vi "Actor Core.vi"(8 "error in":errorcluster, 11 "KIT-QA in":refnum<class "KIT-QA.lvclass">) -> (0 "error out":errorcluster, 3 "Actor out":refnum<class "Actor.lvclass">)   [LabVIEW 2015, in "KIT-QA.lvlib" / "KIT-QA.lvclass"]
doc: "(<B>Filename</B>: Actor Framework.lvlib:Actor.lvclass:Actor Core.vi)\n\nReceives messages to the actor, reacts to them, and initiates any error handling that may shut the actor down.\n\nDescendant classes may override this VI to append parallel tasks for the actor to complete while it handles messages. Overrides use the Call Parent Method node."
uses:
  KIT-QA.lvclass
  <vilib>/ActorFramework/Actor/Actor.lvclass
  CSPP_Core/Actors/CS++BaseActor/CS++BaseActor.lvclass/CS++BaseActor.ctl
  KIT-QA.lvclass/KIT-QA.ctl
  CSPP_Core/Actors/CS++GUIActor/CS++GUIActor.lvclass/CS++GUIActor.ctl
  <vilib>/ActorFramework/Actor/Actor.lvclass/Actor.ctl
  <vilib>/ActorFramework/Message Enqueuer/Message Enqueuer.lvclass/Message Enqueuer.ctl
  KIT-QA Messages/Save to TDMS Msg/Save to TDMS Msg.lvclass/Save to TDMS Msg.ctl
  KIT-QA Messages/Read QDEvent Logfile Msg/Read QDEvent Logfile Msg.lvclass/Read QDEvent Logfile Msg.ctl
  CSPP_Core/Actors/CS++BaseActor/Read Object Name.vi
  CSPP_Core/Actors/CS++GUIActor/Read Stop-Event.vi
  CSPP_Core/Actors/CS++GUIActor/Read PV-Update.vi
  <vilib>/ActorFramework/Message Enqueuer/Init from Existing Queue.vi
  <vilib>/ActorFramework/Message Enqueuer/Enqueue.vi
  <vilib>/ActorFramework/Message Priority Queue/Priority Enqueue.vi
  <vilib>/Waveform/WDTOps.llb/WDT Waveform Duration DBL.vi
  CSPP_Core/Classes/CS++ProcessVariables/ProcessVariable/PV.lvclass
  <vilib>/ActorFramework/Message Enqueuer/Message Enqueuer.lvclass
  <vilib>/ActorFramework/Stop Msg/Stop Msg.lvclass
  KIT-QA Messages/Save to TDMS Msg/Save to TDMS Msg.lvclass
  KIT-QA Messages/Read QDEvent Logfile Msg/Read QDEvent Logfile Msg.lvclass
  CSPP_Core/Actors/CS++GUIActor/CS++GUIActor.lvclass
  CSPP_Core/Actors/CS++BaseActor/CS++BaseActor.lvclass
  CSPP_Core/Libraries/Utilities/CS++Utilities.lvlib
panel:
  out "Enabled Plots":bool[](array[boolean])
  out "CursLoc":cluster{"X":dbl, "Y":dbl}
  out "Quench Channel":i32
  out "Quench Event Logfile Content":string
  in  "Stop Button":bool
  out "Mixed Signal Graph":T1(graph)
  out "Trace Graph":T2(graph)
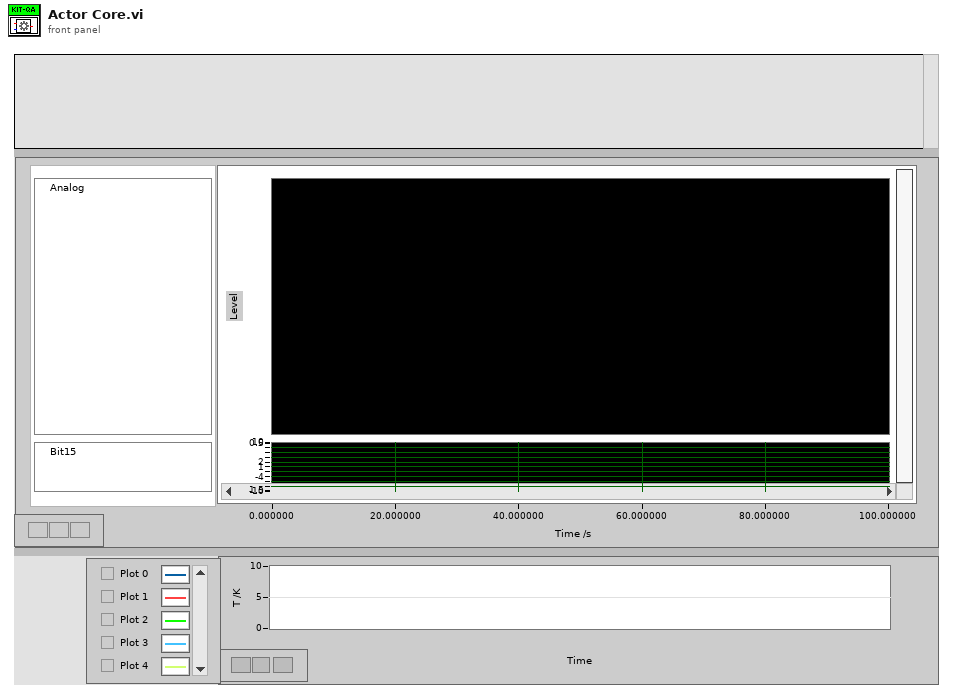
[diagram p1: front panel]
types:
  T1 = cluster{"Analog Wfm":waveform(dbl)[], "Bit 15":digitalwaveform}
  T2 = cluster{"timestamps":timestamp[], "data":dbl[]}[]
  T3 = enum32{"Invalid", "Standard", "Closed", "Hidden", "Minimized", "Maximized"}
  T4 = cluster{"Quench Offset":dbl[unit], "Quench Channel":i32, "Bit 15":digitalwaveform, "Analog Wfm":waveform(dbl)[]}
  T5 = enum8{"Enabled", "Disabled", "Disabled and Grayed Out"}
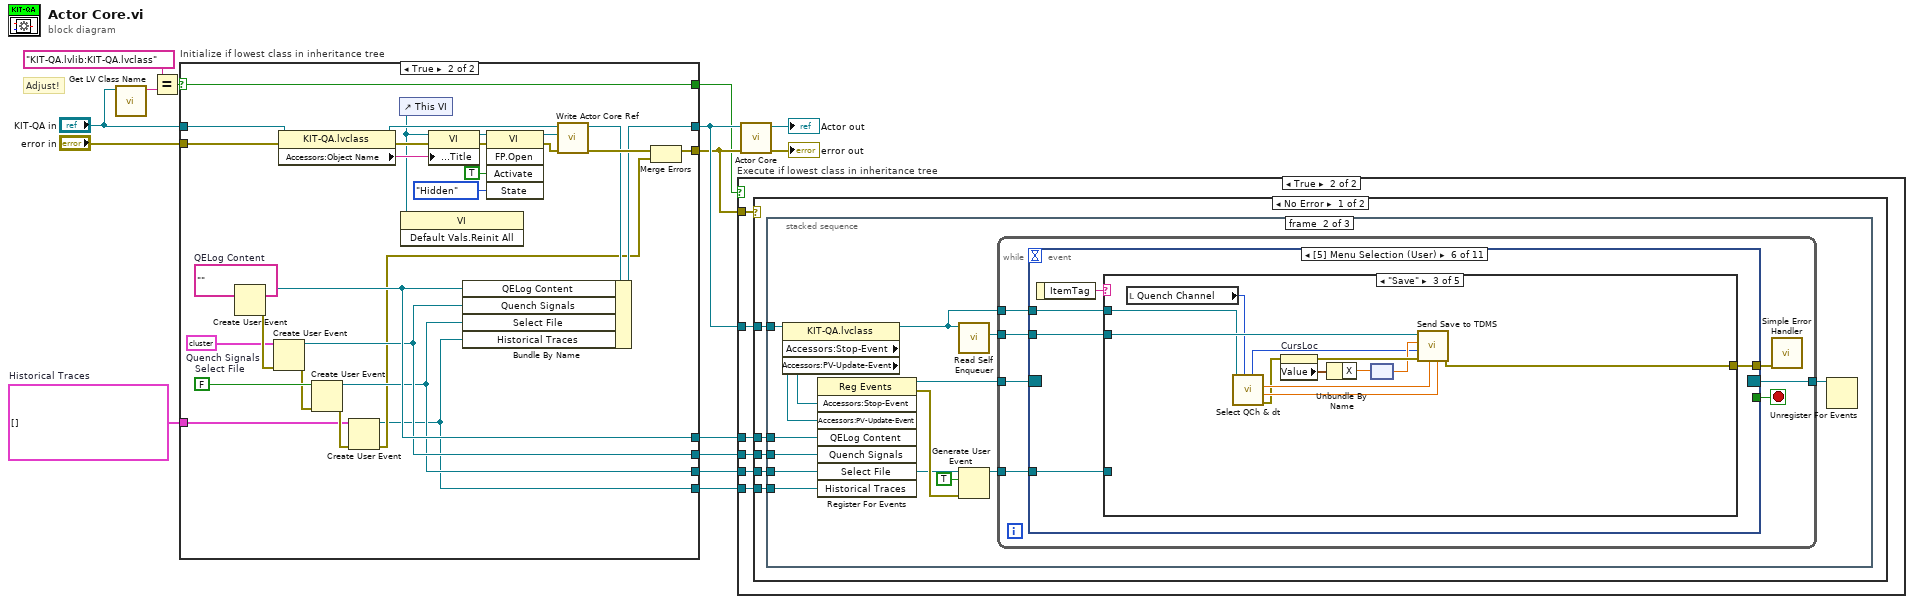
[diagram p0: block diagram]
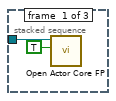
[diagram p3: hidden frame]
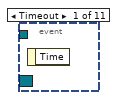
[diagram p4: hidden frame]
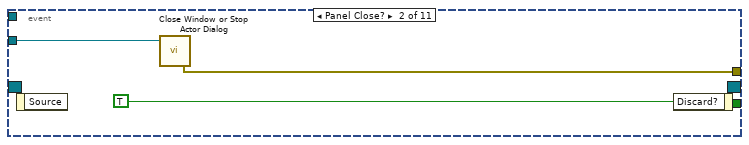
[diagram p5: hidden frame]
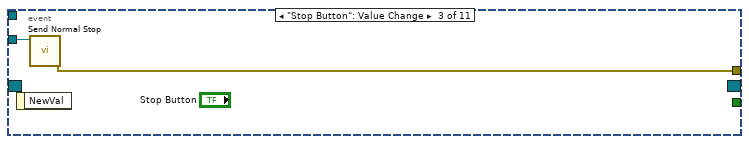
[diagram p6: hidden frame]
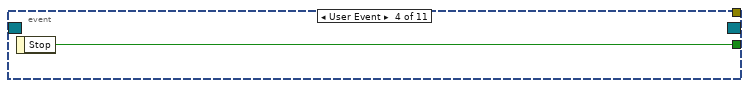
[diagram p7: hidden frame]
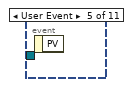
[diagram p8: hidden frame]
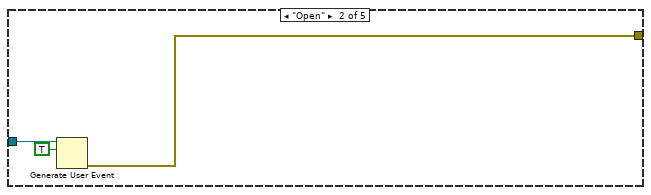
[diagram p10: hidden frame]
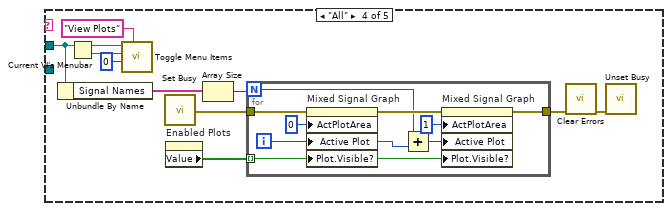
[diagram p11: hidden frame]
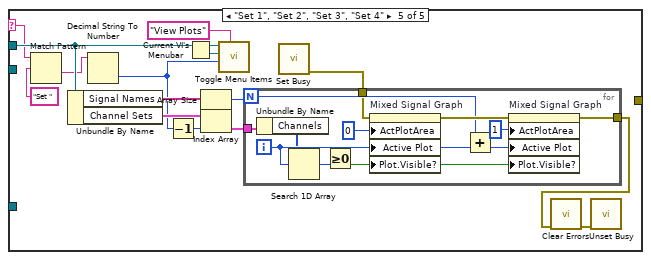
[diagram p12: hidden frame]
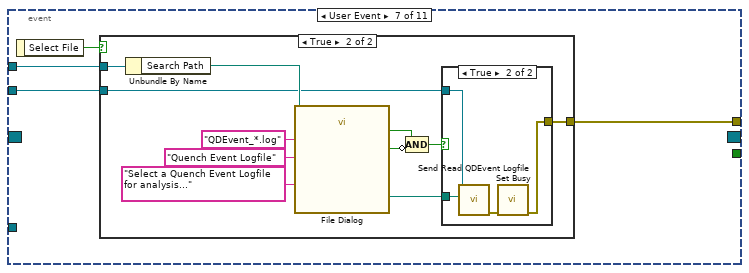
[diagram p13: hidden frame]
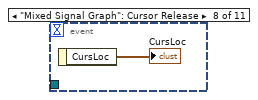
[diagram p16: hidden frame]
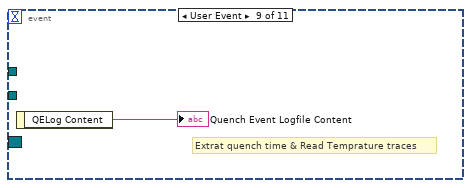
[diagram p17: hidden frame]
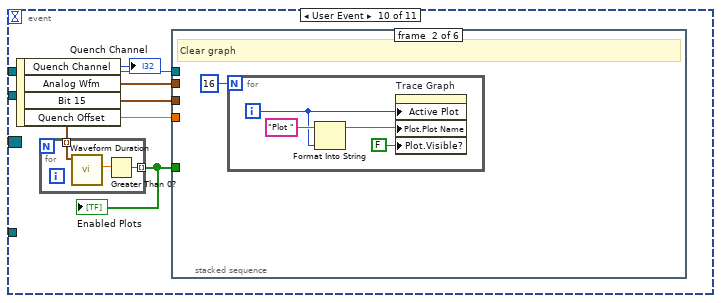
[diagram p18: hidden frame]
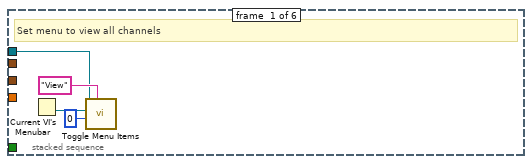
[diagram p19: hidden frame]
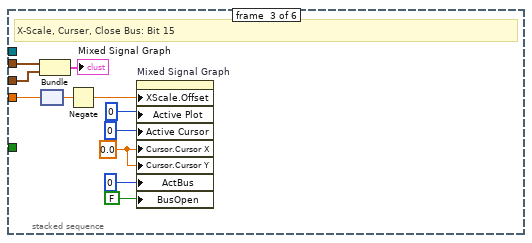
[diagram p20: hidden frame]
diagram:
  w2 = T2 []  # Historical Traces
  # "Adjust!"
  n1 = call <vilib>:"Get LV Class Name.vi"("object"="KIT-QA in") -> ("class name"=w15:string)  [unwired: 9 in, 1 out]
  n2 = Equal?(x="KIT-QA.lvlib:KIT-QA.lvclass" ("class name"), y=w15) -> (x = y?=w11:bool)
  n3 = case "Initialize if lowest class in inheritance tree" shown="True" w11 {
    selector: w11 -> [w18 w45]
    tunnel: "error in" -> [w16 w43]
    tunnel: "KIT-QA in" -> [w17 w28]
    tunnel: [w17 w33] -> w13
    tunnel: [w16 w31] -> w12
    tunnel: [w18 w45] -> w10
    tunnel: [_ w32] -> w5
    tunnel: [_ w29] -> w4
    tunnel: [_ w23] -> w3
    tunnel: w2 -> [_ w20]
    tunnel: [_ w19] -> w1
    frame False {
    }
    frame True {
      w25 = FALSE  # Select File
      w27 = T4 {"Quench Offset"=0.0, "Quench Channel"=0, "Bit 15"={"t0"=timestamp(0 s since 1904-01-01), "dt"=0.0, "Y"={"transitions"=[], "data"=[]}}, "Analog Wfm"=[]}  # Quench Signals
      w35 = ""  # QELog Content
      n4 = Create User Event(user event datatype=w35) -> (user event=w32:refnum<user-event>, error out=w30:errorcluster)  [unwired: 1 in]
      n5 = Create User Event(user event datatype=w27, error in=w30) -> (user event=w29:refnum<user-event>, error out=w24:errorcluster)
      n6 = property class="KIT-QA.lvclass"(reference=w28, error in=w43) -> (reference out=w36:refnum<class "KIT-QA.lvclass">, error out=w38:errorcluster, "Accessors:Object Name"=w37:string)
      n7 = Create User Event(user event datatype=w25, error in=w24) -> (user event=w23:refnum<user-event>, error out=w22:errorcluster)
      n8 = Create User Event(user event datatype=w20, error in=w22) -> (user event=w19:refnum<user-event>, error out=w21:errorcluster)
      n9 = control-ref of="This VI"() -> (w26:refnum<vi>)
      n10 = invoke class="VI" method="Default Vals.Reinit All"(reference=w26) -> ()  [unwired: 2 in, 3 out]
      n11 = property class="VI"(reference=w26, error in=w38, "Front Panel.Title"=w37) -> (reference out=w40:refnum<vi>, error out=w39:errorcluster)
      n12 = invoke class="VI" method="FP.Open"(reference=w40, error in=w39, "Activate"=TRUE ("Activate?"), "State"=T3."Hidden") -> (reference out=w44:refnum<vi>, error out=w42:errorcluster)  [unwired: 1 in, 3 out]
      n13 = call "Write Actor Core Ref.vi"("error in (no error)"=w42, "Actor Core Ref"=w44, "CS++BaseActor in"=w36) -> ("error out"=w41:errorcluster, "CS++BaseActor out"=w34:refnum<class "KIT-QA.lvclass">)  [unwired: 7 in]
      n14 = Bundle By Name(cluster=w34, "QELog Content"=w32, "Quench Signals"=w29, "Select File"=w23, "Historical Traces"=w19) -> (w33:refnum<class "KIT-QA.lvclass">)
      n15 = Merge Errors(w41, w21) -> (w31:errorcluster)
    }
  }
  n16 = case "Execute if lowest class in inheritance tree" shown="True" w10 {
    tunnel: w13 -> [_ w53]
    tunnel: w12 -> [_ w52]
    tunnel: w5 -> [_ w51]
    tunnel: w4 -> [_ w50]
    tunnel: w3 -> [_ w49]
    tunnel: w1 -> [_ w48]
    frame False {
    }
    frame True {
      n17 = case shown="No Error" w52 {
        tunnel: w53 -> [w58 _]
        tunnel: w51 -> [w57 _]
        tunnel: w50 -> [w56 _]
        tunnel: w49 -> [w55 _]
        tunnel: w48 -> [w54 _]
        frame No Error {
          n18 = stacked-sequence {
            tunnel: w58 -> [w60 w74 w247]
            tunnel: w57 -> [_ w68 _]
            tunnel: w56 -> [_ w66 _]
            tunnel: w55 -> [_ w64 _]
            tunnel: w54 -> [_ w61 _]
            frame #0 {
              n19 = call "Open Actor Core FP.vi"("Open FP (F)"=TRUE, "CS++BaseActor in"=w60) -> ()  [unwired: 8 in, 2 out]
            }
            frame #1 {
              n20 = property class="KIT-QA.lvclass"(reference=w74) -> (reference out=w67:refnum<class "KIT-QA.lvclass">, "Accessors:Stop-Event"=w70:refnum<user-event>, "Accessors:PV-Update-Event"=w69:refnum<user-event>)  [unwired: 1 in, 1 out]
              n21 = register-events(w70, w69, w68, w66, w64, w61) -> (reference out=w71:refnum<event-registration>, error out=w65:errorcluster)  [unwired: 2 in]
              n22 = call <vilib>:"Read Self Enqueuer.vi"("Actor"=w67) -> ("Self Enqueuer"=w72:refnum<class "Message Enqueuer.lvclass">)  [unwired: 10 in]
              n23 = Generate User Event(user event=w64, event data cluster=TRUE ("event data"), error in=w65) -> (user event out=w62:refnum<user-event>)  [unwired: 1 in, 1 out]
              n24 = while {
                tunnel: w71 -> [w81]
                tunnel: [w79] -> w73
                tunnel: w72 -> [w77]
                tunnel: w67 -> [w76]
                tunnel: w62 -> [w75]
                stop <- w80 stop-if-true
                n25 = event shown="[5] Menu Selection (User)" {
                  selector: w81 -> [_ _ _ _ _ _ _ _ _ _ _]
                  dyn-events: [_ _ _ _ _ _ _ _ _ _ _] -> w79
                  timeout: _ -> [_ _ _ _ _ _ _ _ _ _ _]
                  tunnel: [_ _ _ w87 _ _ _ _ _ _ _] -> w80
                  tunnel: [_ w82 w86 _ _ w89 w155 _ _ _ _] -> w78
                  tunnel: w77 -> [_ w83 w85 _ _ w90 w157 _ _ _ _]
                  tunnel: w76 -> [_ _ _ _ _ w91 w156 _ _ w179 w230]
                  tunnel: w75 -> [_ _ _ _ _ w88 _ _ _ _ _]
                  event Timeout {
                    n26 = event-data() -> ()  [unwired: 1 in, 1 out]
                  }
                  event Panel Close? {
                    n27 = event-data() -> ()  [unwired: 1 in, 1 out]
                    n28 = call "Close Window or Stop Actor Dialog.vi"("Self Enqueuer"=w83) -> ("Error Out"=w82:errorcluster)  [unwired: 2 in]
                    n29 = event-data("Discard?"=TRUE) -> ()  [unwired: 1 in, 1 out]
                  }
                  event "Stop Button": Value Change {
                    n30 = event-data() -> ()  [unwired: 1 in, 1 out]
                    n31 = call <vilib>:"Send Normal Stop.vi"("Message Enqueuer"=w85) -> ("error out"=w86:errorcluster)  [unwired: 10 in]
                  }
                  event User Event {
                    n32 = event-data() -> ("Stop"=w87:bool)  [unwired: 1 in]
                  }
                  event User Event {
                    n33 = event-data() -> ()  [unwired: 1 in, 1 out]
                  }
                  event Menu Selection (User) {
                    n34 = event-data() -> ("ItemTag"=w92:string)  [unwired: 1 in]
                    n35 = case shown="\"Save\"" w92 {
                      selector: w92 -> [_ _ _ _ w135]
                      tunnel: w91 -> [_ _ w101 w114 w139]
                      tunnel: w90 -> [_ _ w107 _ _]
                      tunnel: [_ w93 w106 _ _] -> w89
                      tunnel: w88 -> [_ w94 _ _ _]
                      frame "False", Default {
                      }
                      frame "Open" {
                        n36 = Generate User Event(user event=w94, event data cluster=TRUE ("event data")) -> (error out=w93:errorcluster)  [unwired: 2 in, 1 out]
                      }
                      frame "Save" {
                        n37 = local read "Quench Channel"() -> (w100:i32)
                        n38 = call "Select QCh & dt.vi"("Quench Channel in"=w100, "KIT-QA in"=w101) -> ("Error Out"=w96:errorcluster, "Stop Time out"=w97:dbl[unit], "Start Time out"=w98:dbl[unit], "Quench Channel out"=w99:i32)  [unwired: 5 in, 1 out]
                        n39 = property on="CursLoc" class="Clust (strict)"(error in=w96) -> (error out=w105:errorcluster, "Value"=w104:cluster{"X":dbl, "Y":dbl})  [unwired: 1 in, 1 out]
                        n40 = Unbundle By Name(w104) -> ("X"=w103:dbl)
                        n41 = node(w103) -> (w102:dbl[unit])
                        n42 = call "Send Save to TDMS.vi"("Stop Time"=w97, "Start Time"=w98, "error in (no error)"=w105, "Quench Channel"=w99, "Quench Start"=w102, "Message Enqueuer"=w107) -> ("error out"=w106:errorcluster)  [unwired: 4 in, 1 out]
                      }
                      frame "All" {
                        n43 = Unbundle By Name(w114) -> ("Signal Names"=w112:string[])
                        n44 = Current VI's Menubar() -> (w116:refnum<k9>)
                        n45 = call "Toggle Menu Items.vi"("Item Tag"="View Plots" ("item tag"), "Item Index"=0, "Menu Ref"=w116, "KIT-QA in"=w114) -> ()  [unwired: 6 in, 2 out]
                        n46 = call <vilib>:"Set Busy.vi"() -> ("error out"=w110:errorcluster)  [unwired: 10 in, 1 out]
                        n47 = property on="Enabled Plots" class="Arr (strict)"() -> ("Value"=w111:bool[])  [unwired: 2 in, 2 out]
                        n48 = Array Size(array=w112) -> (size(s)=w113:i32)
                        n49 = for {
                          N: w113 -> [w121]
                          tunnel: w111 -> [w120] mode=indexing
                          tunnel: w110 -> [w119]
                          tunnel: [w118] -> w109
                          i -> [w123]
                          n50 = property on="Mixed Signal Graph" class="MixedGraph (strict)"(error in=w119, "ActPlotArea"=0 ("Active Plot Area"), "Active Plot"=w123, "Plot.Visible?"=w120) -> (error out=w124:errorcluster)  [unwired: 1 in, 1 out]
                          n51 = Add(x=w121, y=w123) -> (x+y=w122:i32)
                          n52 = property on="Mixed Signal Graph" class="MixedGraph (strict)"(error in=w124, "ActPlotArea"=1 ("Active Plot Area"), "Active Plot"=w122, "Plot.Visible?"=w120) -> (error out=w118:errorcluster)  [unwired: 1 in, 1 out]
                        }
                        n53 = call <vilib>:"Clear Errors.vi"("error in (no error)"=w109) -> ("error out"=w108:errorcluster)  [unwired: 5 in, 1 out]
                        n54 = call <vilib>:"Unset Busy.vi"("error in (no error)"=w108) -> ()  [unwired: 10 in, 1 out]
                      }
                      frame "Set 1", "Set 2", "Set 3", "Set 4" {
                        n55 = Match Pattern(string=w135, regular expression="Set ") -> (after substring=w133:string)  [unwired: 1 in, 3 out]
                        n56 = Unbundle By Name(w139) -> ("Signal Names"=w137:string[], "Channel Sets"=w136:cluster{"Channels":i32[]}[])
                        n57 = Decimal String To Number(string=w133) -> (number=w131:i32)  [unwired: 2 in, 1 out]
                        n58 = Decrement(x=w131) -> (x-1=w130:i32)
                        n59 = Current VI's Menubar() -> (w140:refnum<k9>)
                        n60 = Array Size(array=w137) -> (size(s)=w138:i32)
                        n61 = Index Array(array=w136, index=w130) -> (element=w132:cluster{"Channels":i32[]})
                        n62 = call "Toggle Menu Items.vi"("Item Tag"="View Plots" ("item tag"), "Item Index"=w131, "Menu Ref"=w140, "KIT-QA in"=w139) -> ()  [unwired: 6 in, 2 out]
                        n63 = call <vilib>:"Set Busy.vi"() -> ("error out"=w129:errorcluster)  [unwired: 10 in, 1 out]
                        n64 = for {
                          N: w138 -> [w144]
                          tunnel: w132 -> [w147]
                          tunnel: w129 -> [w143]
                          tunnel: [w142] -> w127
                          i -> [w149]
                          n65 = Unbundle By Name(w147) -> ("Channels"=w146:i32[])
                          n66 = Search 1D Array(1D array=w146, element=w149) -> (index of element=w152:i32)  [unwired: 1 in]
                          n67 = Greater Or Equal To 0?(x=w152) -> (x >= 0?=w148:bool)
                          n68 = property on="Mixed Signal Graph" class="MixedGraph (strict)"(error in=w143, "ActPlotArea"=0 ("Active Plot Area"), "Active Plot"=w149, "Plot.Visible?"=w148) -> (error out=w151:errorcluster)  [unwired: 1 in, 1 out]
                          n69 = Add(x=w144, y=w149) -> (x+y=w145:i32)
                          n70 = property on="Mixed Signal Graph" class="MixedGraph (strict)"(error in=w151, "ActPlotArea"=1 ("Active Plot Area"), "Active Plot"=w145, "Plot.Visible?"=w148) -> (error out=w142:errorcluster)  [unwired: 1 in, 1 out]
                        }
                        n71 = call <vilib>:"Clear Errors.vi"("error in (no error)"=w127) -> ("error out"=w128:errorcluster)  [unwired: 5 in, 1 out]
                        n72 = call <vilib>:"Unset Busy.vi"("error in (no error)"=w128) -> ()  [unwired: 10 in, 1 out]
                      }
                    }
                  }
                  event User Event {
                    n73 = event-data() -> ("Select File"=w154:bool)  [unwired: 1 in]
                    n74 = case shown="True" w154 {
                      tunnel: w157 -> [_ w160]
                      tunnel: w156 -> [_ w159]
                      tunnel: [_ w158] -> w155
                      frame False {
                      }
                      frame True {
                        n75 = Unbundle By Name(w159) -> ("Search Path"=w168:path)
                        n76 = call "File Dialog"("start path"=w168, "prompt"="Select a Quench Event Logfile for analysis...", "pattern (all files)"="QDEvent_*.log", "pattern label"="Quench Event Logfile") -> ("selected path"=w161:path, "exists"=w164:bool, "cancelled"=w163:bool)  [unwired: 8 in, 1 out]
                        n77 = Compound Arithmetic op=AND(w164, invert w163) -> (w162:bool)
                        n78 = case shown="True" w162 {
                          tunnel: w160 -> [_ w172]
                          tunnel: w161 -> [_ w171]
                          tunnel: [_ w169] -> w158
                          frame False {
                          }
                          frame True {
                            n79 = call "Send Read QDEvent Logfile.vi"("Quench Event Logfile"=w171, "Message Enqueuer"=w172) -> ("error out"=w170:errorcluster)  [unwired: 8 in, 1 out]
                            n80 = call <vilib>:"Set Busy.vi"("error in (no error)"=w170) -> ("error out"=w169:errorcluster)  [unwired: 9 in, 1 out]
                          }
                        }
                      }
                    }
                  }
                  event "Mixed Signal Graph": Cursor Release {
                    n81 = event-data() -> ("CursLoc"=→"CursLoc":cluster{"X":dbl, "Y":dbl})  [unwired: 1 in]
                  }
                  event User Event {
                    # "Extrat quench time & Read Temprature traces"
                    n82 = event-data() -> ("QELog Content"=→"Quench Event Logfile Content":string)  [unwired: 1 in]
                  }
                  event User Event {
                    n83 = event-data() -> ("Quench Channel"=→"Quench Channel":i32, "Analog Wfm"=w175:waveform(dbl)[], "Bit 15"=w178:digitalwaveform, "Quench Offset"=w180:dbl[unit])  [unwired: 1 in]
                    n84 = for {
                      tunnel: [w182] -> w177 mode=indexing
                      tunnel: w175 -> [w181] mode=indexing
                      n85 = call-poly <vilib>:"Waveform Duration.vi"("waveform in"=w181) -> ("duration"=w183:dbl)  [unwired: 8 in, 2 out]
                      n86 = Greater Than 0?(x=w183) -> (x > 0?=w182:bool)
                    }
                    "Enabled Plots" <- w177
                    n87 = stacked-sequence {
                      tunnel: w180 -> [_ _ w203 _ _ _]
                      tunnel: w179 -> [w186 _ _ w206 w216 _]
                      tunnel: w175 -> [_ _ w193 _ _ _]
                      tunnel: w178 -> [_ _ w194 _ _ _]
                      tunnel: w177 -> [_ _ _ w204 w213 _]
                      frame #0 {
                        # "Set menu to view all channels"
                        n88 = Current VI's Menubar() -> (w185:refnum<k9>)
                        n89 = call "Toggle Menu Items.vi"("Item Tag"="View" ("item tag"), "Item Index"=0, "Menu Ref"=w185, "KIT-QA in"=w186) -> ()  [unwired: 6 in, 2 out]
                      }
                      frame #1 {
                        # "Clear graph"
                        n90 = for {
                          N: 16 -> [_]
                          i -> [w190]
                          n91 = Format Into String(initial string="Plot ", w190) -> (resulting string=w189:string)  [unwired: 2 in, 1 out]
                          n92 = property on="Trace Graph" class="XYGraph (strict)"("Active Plot"=w190, "Plot.Plot Name"=w189, "Plot.Visible?"=FALSE ("Plot.Visible")) -> ()  [unwired: 2 in, 2 out]
                        }
                      }
                      frame #2 {
                        w195 = 0.0 ("Cursor.Cursor Position:Cursor X")
                        # "X-Scale, Curser, Close Bus: Bit 15"
                        n93 = Bundle("Analog Wfm"=w193, "Bit 15"=w194) -> (→"Mixed Signal Graph":T1)  [unwired: 1 in]
                        n94 = node(w203) -> (w202:dbl)
                        n95 = Negate(x=w202) -> (-x=w201:dbl)
                        n96 = property on="Mixed Signal Graph" class="MixedGraph (strict)"("XScale.Offset"=w201, "Active Plot"=u32 0, "Active Cursor"=u32 0, "Cursor.Cursor X"=w195, "Cursor.Cursor Y"=w195, "ActBus"=u32 0 ("Active Plot"), "BusOpen"=FALSE ("Bus Open")) -> ()  [unwired: 2 in, 2 out]
                      }
                      frame #3 {
                        # "Analog signal names"
                        n97 = Unbundle By Name(w206) -> ("Signal Names"=w205:string[])
                        n98 = for {
                          tunnel: w205 -> [w210] mode=indexing
                          tunnel: w204 -> [w207] mode=indexing
                          i -> [w211]
                          n99 = Empty String/Path?(string/path=w210) -> (empty?=w209:bool)
                          n100 = Compound Arithmetic op=AND(invert w209, w207) -> (w208:bool)
                          n101 = property on="Mixed Signal Graph" class="MixedGraph (strict)"("ActPlotArea"=0 ("Active Plot Area"), "Active Plot"=w211, "Plot.Plot Name"=w210, "Plot.Visible?"=w208) -> ()  [unwired: 2 in, 2 out]
                        }
                      }
                      frame #4 {
                        # "Bit 15 signal names"
                        n102 = Unbundle By Name(w216) -> ("Signal Names"=w214:string[])
                        n103 = Array Size(array=w214) -> (size(s)=w215:i32)
                        n104 = for {
                          tunnel: w214 -> [w222] mode=indexing
                          tunnel: w215 -> [w220]
                          tunnel: w213 -> [w217] mode=indexing
                          i -> [w223]
                          n105 = Empty String/Path?(string/path=w222) -> (empty?=w218:bool)
                          n106 = Add(x=w220, y=w223) -> (x+y=w221:i32)
                          n107 = Compound Arithmetic op=AND(invert w218, w217) -> (w219:bool)
                          n108 = property on="Mixed Signal Graph" class="MixedGraph (strict)"("ActPlotArea"=1 ("Active Plot Area"), "Active Plot"=w221, "Plot.Plot Name"=w222, "Plot.Visible?"=w219) -> ()  [unwired: 2 in, 2 out]
                        }
                      }
                      frame #5 {
                        # "Unset busy"
                        n109 = call <vilib>:"Unset Busy.vi"() -> ()  [unwired: 11 in, 1 out]
                      }
                    }
                  }
                  event User Event {
                    n110 = event-data() -> ("Historical Traces"=→"Trace Graph":T2)  [unwired: 1 in]
                    n111 = Unbundle By Name(w230) -> ("Trace Names"=w229:refnum<k21>[])
                    n112 = Empty Array?(array=w229) -> (empty?=w225:bool)
                    n113 = case shown="False" w225 {
                      tunnel: w229 -> [w232 _]
                      frame False {
                        n114 = for {
                          tunnel: w232 -> [w239] mode=indexing
                          i -> [w234]
                          n115 = Reverse String(1:w239) -> (0:w238:string)
                          n116 = Match Pattern(string=w238, regular expression="\\\\") -> (before substring=w237:string)  [unwired: 1 in, 3 out]
                          n117 = Reverse String(1:w237) -> (0:w235:string)
                          n118 = property on="Trace Graph" class="XYGraph (strict)"("Active Plot"=w234, "Plot.Plot Name"=w235, "Plot.Visible?"=TRUE ("Plot.Visible")) -> ()  [unwired: 2 in, 2 out]
                        }
                      }
                      frame True {
                      }
                    }
                    n119 = Select(t=T5."Disabled and Grayed Out" ("Disabled"), s=w225, f=T5."Enabled" ("Disabled")) -> (s? t:f=w228:T5)
                    n120 = property on="Trace Graph" class="XYGraph (strict)"("DisabledEnum"=w228) -> ()  [unwired: 2 in, 2 out]
                  }
                }
                n121 = call <vilib>:"Simple Error Handler.vi"("error in (no error)"=w78) -> ()  [unwired: 4 in, 5 out]
              }
              n122 = Unregister For Events(event registration refnum=w73) -> ()  [unwired: 1 in, 1 out]
            }
            frame #2 {
              n123 = call "Open Actor Core FP.vi"("Open FP (F)"=FALSE, "CS++BaseActor in"=w247) -> ("CS++BaseActor out"=w242:refnum<class "KIT-QA.lvclass">)  [unwired: 8 in, 1 out]
              n124 = call-dynamic "Destroy User Define Events.vi"("CS++GUIActor in"=w242) -> ("CS++GUIActor out"=w245:refnum<class "KIT-QA.lvclass">)  [unwired: 9 in, 1 out]
              n125 = Unbundle By Name(w245) -> ("QELog Content"=w244:refnum<user-event>, "Quench Signals"=w243:refnum<user-event>, "Select File"=w241:refnum<user-event>, "Historical Traces"=w240:refnum<user-event>)
              n126 = Destroy User Event(user event=w244) -> ()  [unwired: 1 in, 1 out]
              n127 = Destroy User Event(user event=w243) -> ()  [unwired: 1 in, 1 out]
              n128 = Destroy User Event(user event=w241) -> ()  [unwired: 1 in, 1 out]
              n129 = Destroy User Event(user event=w240) -> ()  [unwired: 1 in, 1 out]
            }
          }
        }
        frame Error {
        }
      }
    }
  }
  n130 = call-parent "Actor Core.vi"("error in"=w12, "CS++GUIActor in"=w13) -> ("error out"=→"error out":errorcluster, "Actor out"=→"Actor out":refnum<class "Actor.lvclass">)  [unwired: 8 in]
